vi "Core Create.vi"(8 "error in (no error)":errorcluster, 10 "Plugin Name":string, 11 "CIFTemplateNode in":refnum<class "CIFCorePlugin.lvclass">) -> (0 "error out":errorcluster, 3 "CIFTemplateNode out":refnum<class "CIFCorePlugin.lvclass">)   [LabVIEW 2021, in "CIFCorePlugin.lvclass"]
uses:
  CIFCorePlugin.lvclass
  Typedef/Energized States.ctl
  Typedef/Log Type.ctl
  OOB/OOB_Rx/CIFCoreOOB_Rx.lvclass/CIFCoreOOB_Rx.ctl
  CIFUtilities/CIFOutOfBand/CIFOutOfBand.lvclass/CIFOutOfBand.ctl
  CIFCorePlugin.lvclass/CIFCorePlugin.ctl
  OOB/OOB_Rx/Private/Command Settings.vi
  CIFUtilities/CIFOutOfBand/Accessors/Write Local OOB Data.vi
  OOB/OOB_Tx/Private/Command Settings.vi
  Accessors/Get Time.vi
  Common/Utilities/Update Delta Time.vi
  Accessors/Timestamps/Read Creation TS.vi
  CIFUtilities/CIFClocks/Core/Get Time.vi
  CIFUtilities/CIFClocks/SubVIs/Add Error.vi
  CIFUtilities/CIFClocks/Time Conversion/LabVIEW Time to UTC Time.vi
  Common/Utilities/Append Error Location.vi
  OOB/OOB_Rx/CIFCoreOOB_Rx.lvclass
  D:/dev/CIF-LVCore/src/CIFUtilities/CIFOutOfBand/CIFOutOfBand.lvclass
  OOB/OOB_Tx/CIFCoreOOB_Tx.lvclass
  CIFUtilities/CIFOutOfBand/Init OOB.vi
  Common/CIFCoreCommon.lvlib
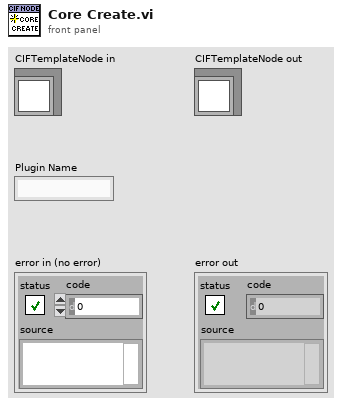
[diagram p1: front panel]
types:
  T1 = typedef "CIFCorePlugin.lvclass/Log Type.ctl" = enum16{"Info", "Config"}
  T2 = typedef "CIFCorePlugin.lvclass/Energized States.ctl" = enum16{"Listen", "Prepare", "Execute", "Housekeep", "Cleanup", "Destroy"}
  T3 = typedef "CIFCoreCommon.lvlib/Version.ctl" = cluster{"Major":i32, "Minor":i32, "Fix":i32, "Build":i32}
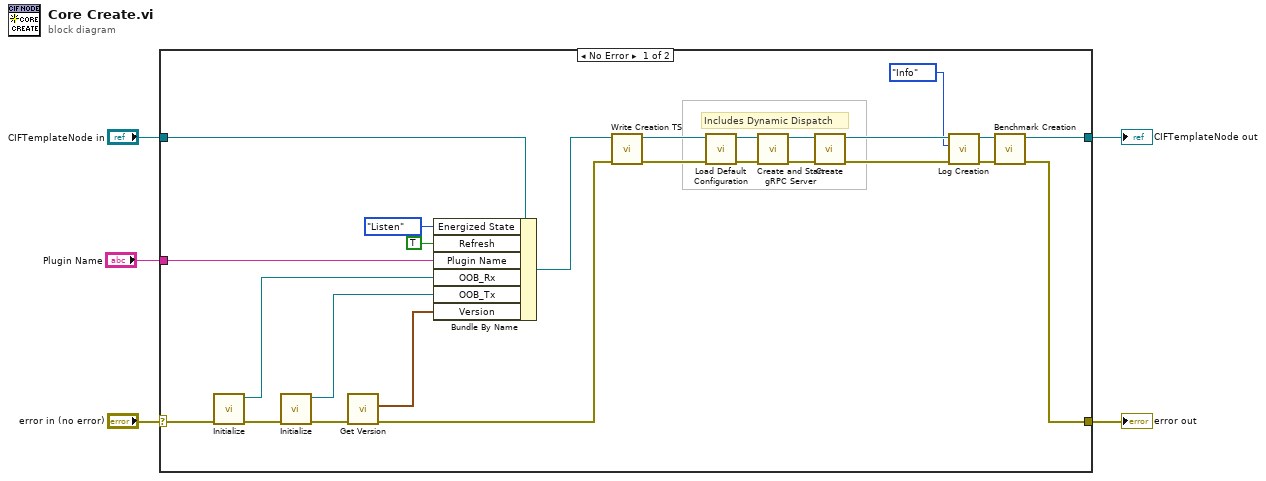
[diagram p0: block diagram]
diagram:
  n1 = case shown="No Error" "error in (no error)" {
    selector: "error in (no error)" -> [w27 w32]
    tunnel: [w12 w32] -> w4
    tunnel: [w13 w31] -> w2
    tunnel: "CIFTemplateNode in" -> [w11 w31]
    tunnel: "Plugin Name" -> [w26 _]
    frame No Error {
      # "Includes Dynamic Dispatch"
      n2 = call "Initialize.vi"("error in"=w27) -> ("error out"=w28:errorcluster, "CoreOOB_Rx out"=w30:refnum<class "CIFCoreOOB_Rx.lvclass">)  [unwired: 9 in]
      n3 = call "Initialize.vi"("error in"=w28) -> ("error out"=w25:errorcluster, "CoreOOB_Tx out"=w29:refnum<class "CIFCoreOOB_Tx.lvclass">)  [unwired: 9 in]
      n4 = call "Get Version.vi"("error in (no error)"=w25) -> ("error out"=w17:errorcluster, "Version"=w24:T3)  [unwired: 9 in]
      n5 = Bundle By Name(cluster=w11, "Energized State"=Energized_States."Listen", "Refresh"=TRUE, "Plugin Name"=w26, "OOB_Rx"=w30, "OOB_Tx"=w29, "Version"=w24) -> (w14:refnum<class "CIFCorePlugin.lvclass">)
      n6 = call "Write Creation TS.vi"("error in (no error)"=w17, "CIFCorePlugin in"=w14) -> ("error out"=w16:errorcluster, "CIFCorePlugin out"=w15:refnum<class "CIFCorePlugin.lvclass">)  [unwired: 8 in]
      n7 = call-dynamic "Load Default Configuration.vi"("error in (no error)"=w16, "CIFTemplateNode in"=w15) -> ("error out"=w23:errorcluster, "CIFTemplateNode out"=w22:refnum<class "CIFCorePlugin.lvclass">)  [unwired: 8 in]
      n8 = call "Create and Start gRPC Server.vi"("error in (no error)"=w23, "CIFTemplateNode in"=w22) -> ("error out"=w20:errorcluster, "CIFTemplateNode out"=w21:refnum<class "CIFCorePlugin.lvclass">)  [unwired: 8 in]
      n9 = call-dynamic "Create.vi"("error in (no error)"=w20, "CIFTemplateNode in"=w21) -> ("error out"=w9:errorcluster, "CIFTemplateNode out"=w10:refnum<class "CIFCorePlugin.lvclass">)  [unwired: 8 in]
      n10 = call "Log Creation.vi"("error in (no error)"=w9, "Log Type"=Log_Type."Info", "CIFCorePlugin in"=w10) -> ("error out"=w8:errorcluster, "CIFCorePlugin out"=w7:refnum<class "CIFCorePlugin.lvclass">)  [unwired: 7 in]
      n11 = call "Benchmark Creation.vi"("error in (no error)"=w8, "CIFCorePlugin in"=w7) -> ("error out"=w12:errorcluster, "CIFCorePlugin out"=w13:refnum<class "CIFCorePlugin.lvclass">)  [unwired: 8 in]
    }
    frame Error {
    }
  }
  "error out" <- w4
  "CIFTemplateNode out" <- w2
